vi "Check User Abort.vi"(8 "error in (no error)":errorcluster) -> (0 "error out":errorcluster)   [LabVIEW 2019, in "ACSVcontrol-driver.lvlib"]
doc: "Checks if boolean Abort is positive and generate user abort error."
uses:
  ACSVcontrol-driver.lvlib
  Globals.vi
  <vilib>/Utility/error.llb/Error Cluster From Error Code.vi
  <vilib>/ErrorRing/Error Ring.xnode
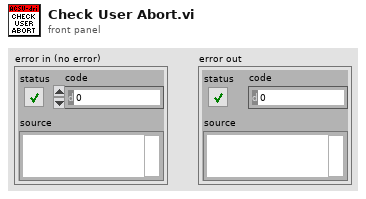
[diagram p1: front panel]
types:
  T1 = enum8{"Enabled", "Disabled", "Disabled and Grayed Out"}
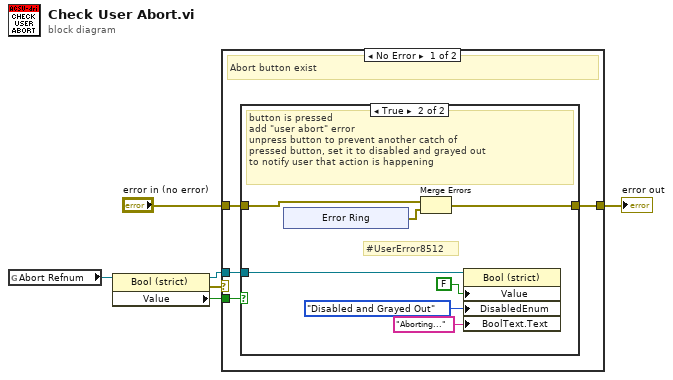
[diagram p0: block diagram]
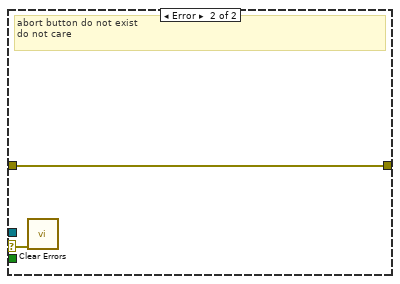
[diagram p3: hidden frame]
diagram:
  n1 = global read "Globals.vi" "Abort Refnum"() -> (w6:refnum<vi>)
  n2 = property class="Bool (strict)"(reference=w6) -> (reference out=w1:refnum<vi>, error out=w5:errorcluster, "Value"=w4:bool)  [unwired: 1 in]
  n3 = case shown="No Error" w5 {
    selector: w5 -> [_ w24]
    tunnel: w4 -> [w7 _]
    tunnel: "error in (no error)" -> [w10 w25]
    tunnel: [w9 w25] -> w2
    tunnel: w1 -> [w8 _]
    frame No Error {
      # "Abort button exist"
      n4 = case shown="True" w7 {
        tunnel: w10 -> [w11 w18]
        tunnel: [w11 w17] -> w9
        tunnel: w8 -> [_ w16]
        frame False {
          # "button not pressed, nothing happens"
        }
        frame True {
          # "#UserError8512"
          # "button is pressed\nadd \"user abort\" error\nunpress button to prevent another catch of \npressed button, set it to disabled and grayed out \nto notify user that action is happening"
          n5 = xnode "Error Ring"() -> ("error out"=w13:errorcluster)
          n6 = Merge Errors(w18, w13) -> (w17:errorcluster)
          n7 = property class="Bool (strict)"(reference=w16, "Value"=FALSE, "DisabledEnum"=T1."Disabled and Grayed Out" ("Disabled"), "BoolText.Text"="Aborting..." ("Boolean Text.Text")) -> ()  [unwired: 1 in, 2 out]
        }
      }
    }
    frame Error {
      # "abort button do not exist\ndo not care"
      n8 = call <vilib>:"Clear Errors.vi"("error in (no error)"=w24) -> ()  [unwired: 5 in, 2 out]
    }
  }
  "error out" <- w2
